vi "Shoot Cube Switch V.3.0.vi"(8 "Input Button":bool, 11 "Time Until Reset":i32) -> (1 "On?":bool)   [LabVIEW 2017]
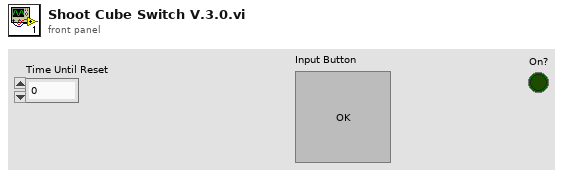
[diagram p1: front panel]
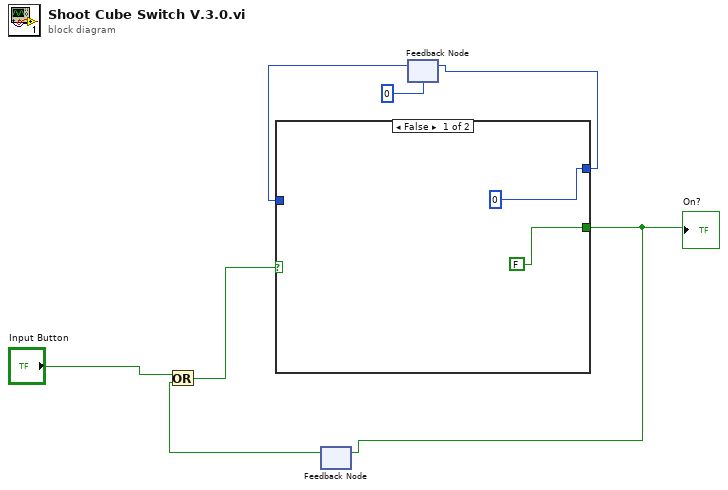
[diagram p0: block diagram]
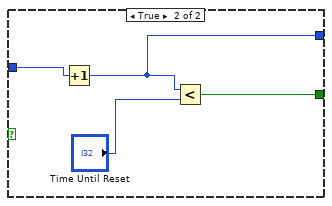
[diagram p2: hidden frame]
diagram:
  n1 = feedback #1() -> (w5:bool)  [unwired: 1 in]
  n2 = Or(x="Input Button", y=w5) -> (x .or. y?=w6:bool)
  n3 = feedback #2(0) -> (w3:i32)
  n4 = case shown="False" w6 {
    tunnel: w3 -> [_ w12]
    tunnel: [0 w11] -> w2
    tunnel: [FALSE w10] -> w1
    frame False {
    }
    frame True {
      n5 = Increment(x=w12) -> (x+1=w11:i32)
      n6 = Less?(x=w11, y="Time Until Reset") -> (x < y?=w10:bool)
    }
  }
  "On?" <- w1
  n7 = feedback-in #1(w1) -> ()
  n8 = feedback-in #2(w2) -> ()
